vi "Get Event Status Register.vi"(8 "error in (no error)":errorcluster, 11 "VISA resource name":refnum<visa-resource-name>) -> (0 "error out":errorcluster, 2 "Event Status Register":bool[](array[boolean]), 3 "VISA resource name out":refnum<visa-resource-name>)   [LabVIEW 2018, in "DPO4104.lvlib" / "DPO4104.lvclass"]
doc: "This VI queries the Event Status Register.\n\nBit 7(MSB) PON Power On. Shows that the oscilloscope was powered on. On completion,the diagnostic self tests also set this bit. \nBit 6 URQ User Request. Indicates that an application event has occurred. \nBit 5 CME Command Error. Shows that an error occurred while the oscilloscope was parsing acommand or query. \nBit 4 EXE Execution Error. Shows that an error executing a command or query. \nBit 3 DDE Device Error. Shows that a device error occurred. \nBit 2 QYE Query Error. Either an attempt was made to read the Output Queue when no data was present or pending, or that data in the Output Queue was lost. \nBit 1 RQC Request Control. This is not used. \nBit 0(LSB) OPC Operation Complete. Shows that the operation is complete. This bit is set when all pending operations complete following an *OPC command."
uses:
  DPO4104.lvclass
  <instrlib>/Tektronix DPO MSO 2000 4000 Series/Tektronix DPO MSO 2000 4000 Series.lvlib
panel:
  # "OPC - Operation Complete"
  # "RQC - Request Control"
  # "QYE  - Query Error"
  # "DDE - DEvice Error"
  # "EXE - Execution Error"
  # "CME - Command Error"
  # "URQ - User  Request"
  # "PON - Power On"
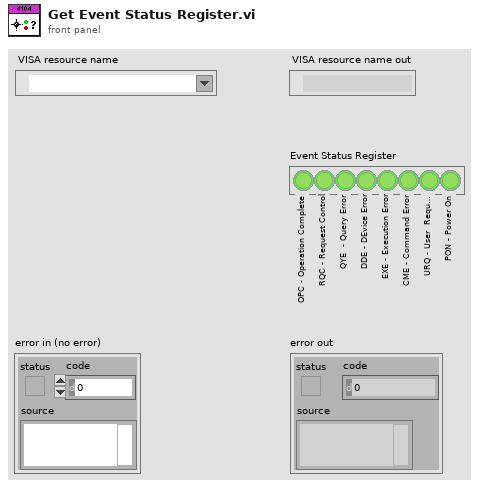
[diagram p1: front panel]
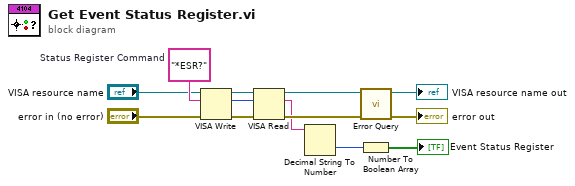
[diagram p0: block diagram]
diagram:
  w9 = "*ESR?"  # Status Register Command
  n1 = VISA Write(VISA resource name="VISA resource name", write buffer=w9, error in (no error)="error in (no error)") -> (VISA resource name out=w13:refnum<visa-resource-name>, return count=w3:u32, error out=w12:errorcluster)
  n2 = VISA Read(VISA resource name=w13, byte count=w3, error in (no error)=w12) -> (VISA resource name out=w6:refnum<visa-resource-name>, read buffer=w4:string, error out=w5:errorcluster)  [unwired: 1 out]
  n3 = Decimal String To Number(string=w4) -> (number=w8:i32)  [unwired: 2 in, 1 out]
  n4 = call <instrlib>:"Error Query.vi"("error in (no error)"=w5, "VISA resource name"=w6) -> ("error out"=→"error out":errorcluster, "VISA resource name out"=→"VISA resource name out":refnum<visa-resource-name>)  [unwired: 6 in, 2 out]
  n5 = Number To Boolean Array(number=w8) -> (Boolean array=→"Event Status Register":bool[])
